vi "SetActualValues.vi"(2 "ActualValues":cluster{"T":dbl, "RH":dbl} {"RH" format="%.2f"; "T" format="%.2f"}, 5 "error in (no error)":errorcluster) -> (19 "error out":errorcluster)   [LabVIEW 2019, in "WebServiceData.lvclass"]
uses:
  WebServiceData.lvclass
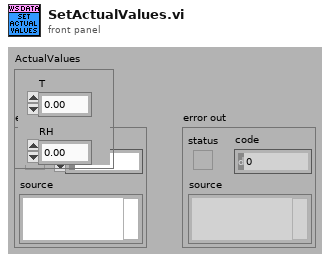
[diagram p1: front panel]
types:
  T1 = typedef "WebServiceData.lvclass/ObjectAttributes.ctl" = cluster{"ActualValues":cluster{"T":dbl, "RH":dbl}}
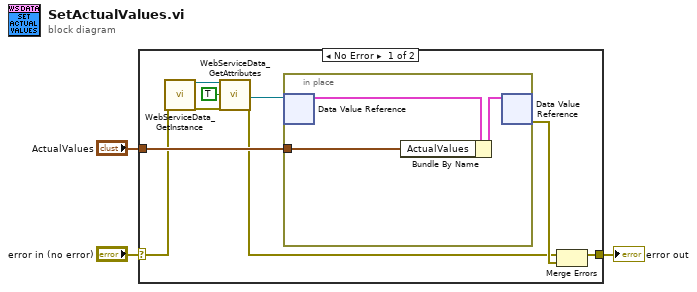
[diagram p0: block diagram]
diagram:
  n1 = case shown="No Error" "error in (no error)" {
    selector: "error in (no error)" -> [w6 w16]
    tunnel: [w10 w16] -> w2
    tunnel: "ActualValues" -> [w12 _]
    frame No Error {
      n2 = call "WebServiceData_GetInstance.vi"("error in (no error)"=w6) -> ("reference out"=w7:refnum<class "WebServiceData.lvclass">, "error out"=w8:errorcluster)  [unwired: 14 in, 3 out]
      n3 = call "WebServiceData_GetAttributes.vi"("reference in"=w7, "OnlyGetDvrReference(False)"=TRUE, "error in (no error)"=w8) -> ("DataRef"=w5:refnum<data-value>, "error out"=w9:errorcluster)  [unwired: 13 in, 2 out]
      n4 = in-place {
        in-place-border: w12 -> [w15]
        n5 = in-place-dvr #1(w5) -> (w14:T1)  [unwired: 1 out]
        n6 = Bundle By Name(cluster=w14, "ActualValues"=w15) -> (w13:T1)
        n7 = in-place-dvr #1(w13) -> (w11:errorcluster)  [unwired: 1 out]
      }
      n8 = Merge Errors(w9, w11) -> (w10:errorcluster)
    }
    frame Error {
    }
  }
  "error out" <- w2
